vi "loadShowHolo.vi"(4 "mainPos":T1={"1_Xcenter"=1140.5, "1_Ycenter"=3.5, "1_Diam. X"=94.5, "1_Diam. Y"=95.5, "1_Form fa."=0.9895287958115183, "1_Xi"=1046.0, "1_Xf"=1235.0, "1_Yi"=99.0, "1_Yf"=-92.0}, 5 "True hologram?":bool, 6 "Python session":refnum<k35>, 7 "Display":u16=1, 8 "error in (no error)":errorcluster, 9 "prev. path":path=path "C:/Users/laboratori/pyHolo/Holograms/Radial_complex.png", 10 "SLM1 cluster":T4={"1_Radio"=enum."No Selection", "1_Trans"=55.688622754491014, "1_Phase"=0.0, "1_HoloCode"="field = rho + 1", "1_Semi"=FALSE, "1_Active"=0, "1_ModType"="_complex", "1_Flip"="no flip", "1_HoloNum"=87.0, "1_key1"="s", "1_value1"=-1, "1_key2"="m+1", "1_value2"=-1, "1_Calibration file"="", "1_SLM brand"=""}, 11 "holoImages":T3={"holoMono"="remote image 000002F649398378", "holo2show in"="remote image 000002F649399088", "holo2slm"="remote image 000002F649397C98"}) -> (0 "error out":errorcluster, 1 "path exist":bool=TRUE, 2 "appended path":path=path "C:/Users/laboratori/pyHolo/Holograms/Radial_complex.png", 3 "holo2show out":T2)   [LabVIEW 2023]
uses:
  <vilib>/vision/Image Controls.llb/IMAQ Image.ctl
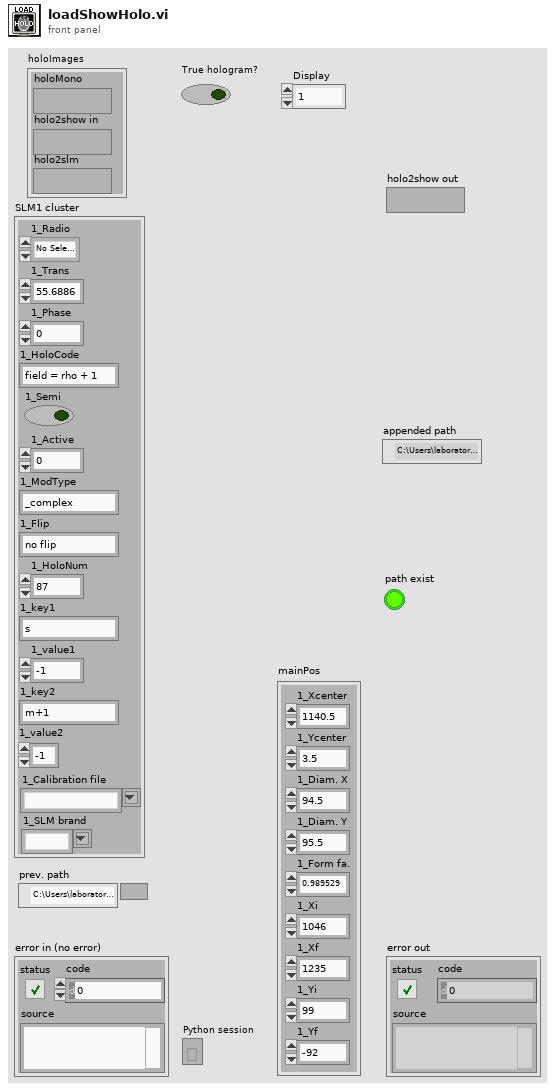
[diagram p1: front panel]
types:
  T1 = cluster{"1_Xcenter":dbl, "1_Ycenter":dbl, "1_Diam. X":dbl, "1_Diam. Y":dbl, "1_Form fa.":dbl, "1_Xi":dbl, "1_Xf":dbl, "1_Yi":dbl, "1_Yf":dbl}
  T2 = typedef "IMAQ Image.ctl" = refnum<image>
  T3 = cluster{"holoMono":T2, "holo2show in":T2, "holo2slm":T2}
  T4 = cluster{"1_Radio":enum32{"No Selection", "Radio Selection 1", "Radio Selection 2", "Radio Selection 3", "Radio Selection 4", "Radio Selection 5", "Radio Selection 6", "Radio Selection 7", "Radio Selection 8"}, "1_Trans":dbl, "1_Phase":dbl, "1_HoloCode":string, "1_Semi":bool, "1_Active":u16, "1_ModType":string, "1_Flip":string, "1_HoloNum":dbl, "1_key1":string, "1_value1":i64, "1_key2":string, "1_value2":i64, "1_Calibration file":string, "1_SLM brand":string}
  T5 = enum32{"No Selection", "Radio Selection 1", "Radio Selection 2", "Radio Selection 3", "Radio Selection 4", "Radio Selection 5", "Radio Selection 6", "Radio Selection 7", "Radio Selection 8"}
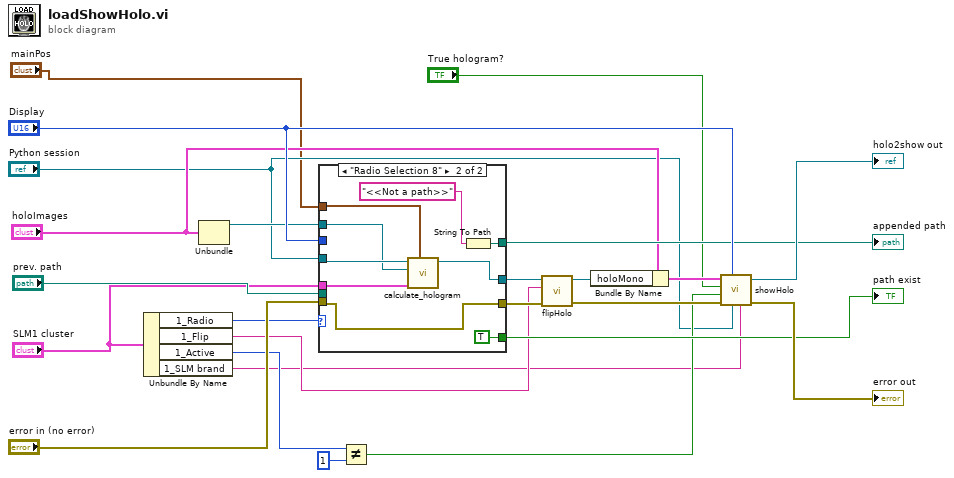
[diagram p0: block diagram]
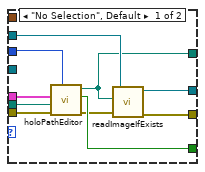
[diagram p2: hidden frame]
diagram:
  n1 = Unbundle By Name("SLM1 cluster") -> ("1_Radio"=w12:T5, "1_Flip"=w13:string, "1_Active"=w11:u16, "1_SLM brand"=w1:string)
  n2 = Unbundle("holoImages") -> ("holoMono"=w8:T2)  [unwired: 2 out]
  n3 = case shown="\"Radio Selection 8\"" w12 {
    tunnel: "prev. path" -> [w34 _]
    tunnel: "error in (no error)" -> [w33 w37]
    tunnel: "Display" -> [w32 _]
    tunnel: "SLM1 cluster" -> [w31 w35]
    tunnel: [w30 w38] -> w17
    tunnel: w8 -> [w29 w42]
    tunnel: [w28 TRUE ("file or folder exists?")] -> w16
    tunnel: [w27 w41] -> w15
    tunnel: [w25 w37] -> w14
    tunnel: "Python session" -> [_ w43]
    tunnel: "mainPos" -> [_ w36]
    frame "No Selection", Default {
      n4 = call "holoPathEditor.vi"("Display"=w32, "error in"=w33, "prev. Path"=w34, "input cluster"=w31) -> ("error out"=w26:errorcluster, "file or folder exists?"=w28:bool, "appended path"=w27:path)  [unwired: 4 in, 1 out]
      n5 = call "readImageIfExists.vi"("error in (no error)"=w26, "appended path"=w27, "Refnum in"=w29) -> ("error out"=w25:errorcluster, "Refnum out"=w30:T2)  [unwired: 7 in]
    }
    frame "Radio Selection 8" {
      n6 = call "calculate_hologram.vi"("mainPos"=w36, "SLM1 cluster"=w35, "monoHolo in"=w42, "pySession"=w43) -> ("monoHolo out"=w38:T2)  [unwired: 7 in]
      n7 = String To Path(string="<<Not a path>>") -> (path=w41:path)
    }
  }
  "appended path" <- w15
  "path exist" <- w16
  n8 = Not Equal?(x=w11, y=u16 1) -> (x != y?=w9:bool)
  n9 = call "flipHolo.vi"("error in (no error)"=w14, "flip_option"=w13, "Image in"=w17) -> ("error out"=w19:errorcluster, "Image out"=w5:T2)  [unwired: 7 in]
  n10 = Bundle By Name(cluster="holoImages", "holoMono"=w5) -> (w7:T3)
  n11 = call "showHolo.vi"("SLM brand"=w1, "pySession"="Python session", "Window Number (0...15)"="Display", "error in (no error)"=w19, "active?"=w9, "True hologram?"="True hologram?", "holoImages"=w7) -> ("error out"=→"error out":errorcluster, "holo2show out"=→"holo2show out":T2)  [unwired: 2 in, 1 out]
